vi "Launch SessionCore.vi"(8 "error in (no error)":errorcluster, 11 "Session in":refnum<class "Session.lvclass">) -> (0 "error out":errorcluster, 2 "Session ID":i32, 3 "Session out":refnum<class "Session.lvclass">)   [LabVIEW 2013, in "MQTT Base.lvlib" / "Session.lvclass"]
uses:
  Session.lvclass
  Session.lvclass/Session.ctl
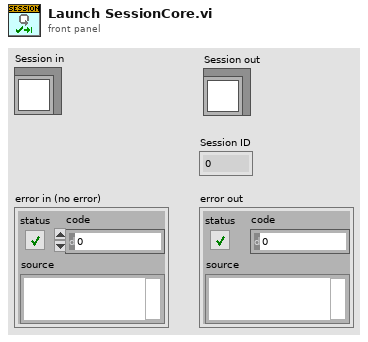
[diagram p1: front panel]
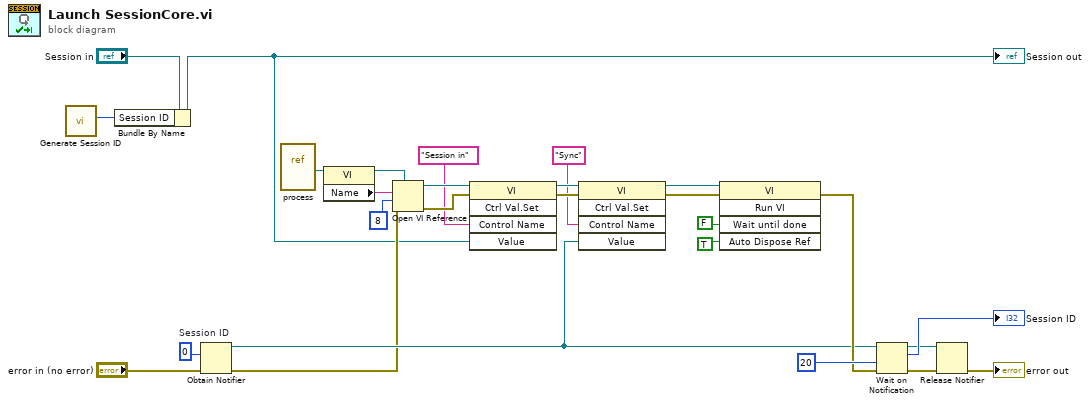
[diagram p0: block diagram]
diagram:
  w21 = 0  # Session ID
  n1 = call "Generate Session ID.vi"() -> ("Session ID"=w3:i32)  [unwired: 11 in]
  n2 = Bundle By Name(cluster="Session in", "Session ID"=w3) -> (w1:refnum<class "Session.lvclass">)
  "Session out" <- w1
  n3 = Obtain Notifier(notification data type=w21, error in (no error)="error in (no error)") -> (notifier out=w19:refnum<notifier>, error out=w4:errorcluster)  [unwired: 2 in, 1 out]
  n4 = vi-ref "process.vi"() -> (w5:refnum<vi>)
  n5 = property class="VI"(reference=w5) -> (reference out=w17:refnum<vi>, "Name"=w18:string)  [unwired: 1 in, 1 out]
  n6 = Open VI Reference(type specifier VI Refnum (for type only)=w17, vi path=w18, options=8, error in (no error)=w4) -> (vi reference=w12:refnum<vi>, error out=w13:errorcluster)  [unwired: 2 in]
  n7 = invoke class="VI" method="Ctrl Val.Set"(reference=w12, error in=w13, "Control Name"="Session in", "Value"=w1) -> (reference out=w10:refnum<vi>, error out=w9:errorcluster)  [unwired: 1 in, 3 out]
  n8 = invoke class="VI" method="Ctrl Val.Set"(reference=w10, error in=w9, "Control Name"="Sync", "Value"=w19) -> (reference out=w7:refnum<vi>, error out=w6:errorcluster)  [unwired: 1 in, 3 out]
  n9 = invoke class="VI" method="Run VI"(reference=w7, error in=w6, "Wait until done"=FALSE ("Wait Until Done"), "Auto Dispose Ref"=TRUE ("Auto Dispose Reference")) -> (error out=w20:errorcluster)  [unwired: 1 in, 4 out]
  n10 = Wait on Notification(notifier=w19, timeout in ms (-1)=20, error in (no error)=w20) -> (notifier out=w22:refnum<notifier>, notification=→"Session ID":i32, error out=w24:errorcluster)  [unwired: 1 in, 1 out]
  n11 = Release Notifier(notifier=w22, error in (no error)=w24) -> (error out=→"error out":errorcluster)  [unwired: 1 in, 2 out]
